vi "MouseclickMultipass.vi"(9 "nMilliseconds":i32=200, 10 "error in (no error)":errorcluster) -> (2 "error out":errorcluster)   [LabVIEW 2014]
panel:
  in  "AutoItX3Lib.IAutoItX3":refnum<k7>
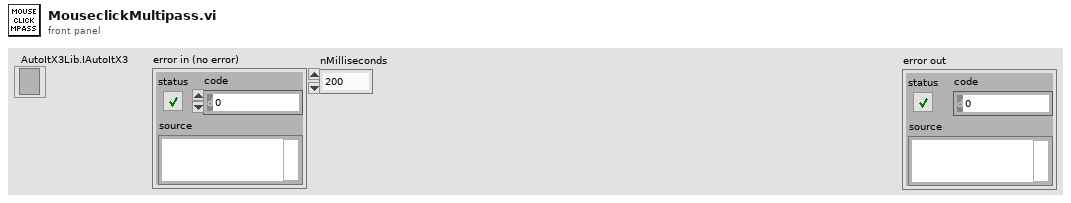
[diagram p1: front panel]
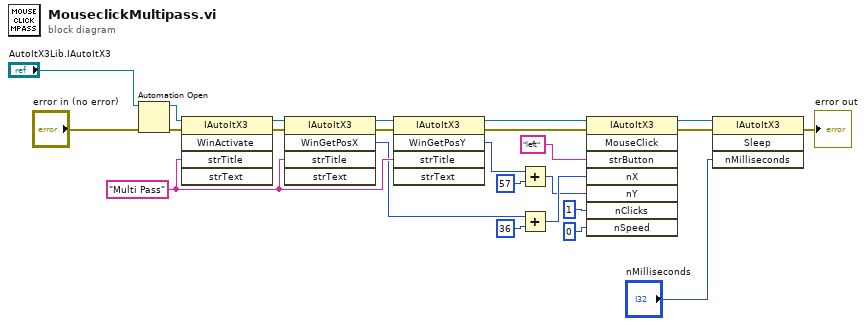
[diagram p0: block diagram]
diagram:
  w12 = "Multi Pass" ("strTitle")
  n1 = Automation Open(error in (no error)="error in (no error)", Automation Refnum="AutoItX3Lib.IAutoItX3") -> (Automation Refnum=w18:refnum<k7>, error out=w17:errorcluster)  [unwired: 2 in]
  n2 = invoke class="IAutoItX3" method="WinActivate"(reference=w18, error in=w17, "strTitle"=w12) -> (reference out=w16:refnum<k7>, error out=w15:errorcluster)  [unwired: 2 in, 3 out]
  n3 = invoke class="IAutoItX3" method="WinGetPosX"(reference=w16, error in=w15, "strTitle"=w12) -> (reference out=w14:refnum<k7>, error out=w13:errorcluster, "WinGetPosX"=w10:i32)  [unwired: 2 in, 2 out]
  n4 = invoke class="IAutoItX3" method="WinGetPosY"(reference=w14, error in=w13, "strTitle"=w12) -> (reference out=w2:refnum<k7>, error out=w1:errorcluster, "WinGetPosY"=w11:i32)  [unwired: 2 in, 2 out]
  n5 = Add(x=w11, y=57) -> (x+y=w4:i32)
  n6 = Add(x=w10, y=36) -> (x+y=w6:i32)
  n7 = invoke class="IAutoItX3" method="MouseClick"(reference=w2, error in=w1, "strButton"="left", "nX"=w6, "nY"=w4, "nClicks"=1, "nSpeed"=0) -> (reference out=w22:refnum<k7>, error out=w21:errorcluster)  [unwired: 1 in, 6 out]
  n8 = invoke class="IAutoItX3" method="Sleep"(reference=w22, error in=w21, "nMilliseconds"="nMilliseconds") -> (error out=→"error out":errorcluster)  [unwired: 1 in, 3 out]
